vi "Configure Averaging.vi"(7 "Enable Averaging (T: Enable)":bool=TRUE, 8 "error in (no error)":errorcluster, 9 "Averaging Count (2)":i32=2 min=2 max=64 step=1, 10 "Averaging Type (0: Exponent)":i32(ring) items=["Exponent", "Linear"], 11 "VISA resource name":refnum<visa-resource-name>) -> (0 "error out":errorcluster, 3 "VISA resource name out":refnum<visa-resource-name>)   [LabVIEW 2021, in "Yokogawa WT1800 Series.lvlib"]
doc: "Configures the averaging features."
uses:
  <instrlib>/Yokogawa WT1800 Series/Yokogawa WT1800 Series.lvlib
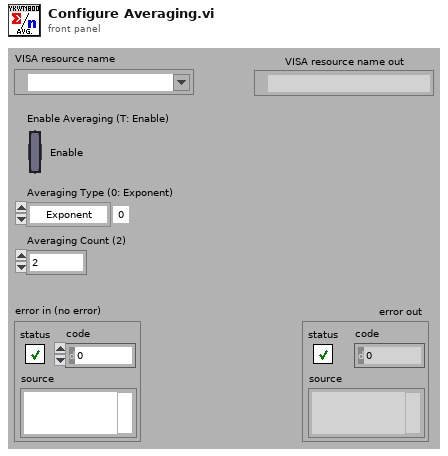
[diagram p1: front panel]
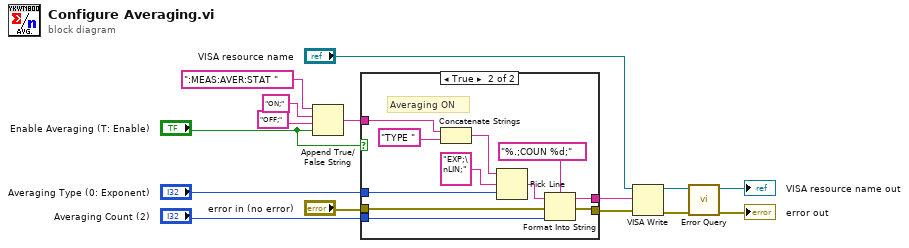
[diagram p0: block diagram]
diagram:
  n1 = Append True/False String ("True/False 文字列を追加")(1:"Enable Averaging (T: Enable)", 2:"OFF;", 3:"ON;", 4:":MEAS:AVER:STAT " ("¶ñi\"\"j")) -> (0:w2:string)
  n2 = case "ケースストラクチャ" shown="True" "Enable Averaging (T: Enable)" {
    tunnel: "Averaging Count (2)" -> [_ w27]
    tunnel: "error in (no error)" -> [w17 w26]
    tunnel: [w16 w25] -> w8
    tunnel: [w17 w18] -> w7
    tunnel: w2 -> [w16 w23]
    tunnel: "Averaging Type (0: Exponent)" -> [_ w20]
    frame False {
      # "Averaging OFF"
    }
    frame True {
      # "Averaging ON"
      n3 = Concatenate Strings(w23, "TYPE ") -> (w21:string)
      n4 = Pick Line ("ライン選択")(string ("")=w21, multi-line string="EXP;\nLIN;" ("複数行文字列"), line index=w20) -> (output string=w19:string)
      n5 = Format Into String ("文字列にフォーマット")(format string="%.;COUN %d;" ("形式文字列"), initial string=w19, error in=w26, w27) -> (resulting string=w25:string, error out=w18:errorcluster)
    }
  }
  n6 = VISA Write ("VISA書き込み")(VISA resource name="VISA resource name", write buffer=w8, error in (no error)=w7) -> (VISA resource name out=w15:refnum<visa-resource-name>, error out=w14:errorcluster)  [unwired: 1 out]
  n7 = call <instrlib>:"Error Query.vi"("error in (no error)"=w14, "VISA resource name"=w15) -> ("error out"=→"error out":errorcluster, "VISA resource name out"=→"VISA resource name out":refnum<visa-resource-name>)  [unwired: 6 in, 2 out]
